vi "open fpga refs.vi"(8 "error in (no error)":errorcluster, 10 "bitfile address":path, 11 "RIO address":string) -> (0 "error out":errorcluster)   [LabVIEW 2014]
uses:
  <vilib>/NI/LVFPGA Adv Session Resources/LVFPGAAdvSessionResources.lvlib
  <vilib>/NI/LVFPGA Adv Session Resources/OpenByName.xnode
  Shared/fpga io types.ctl
  <vilib>/NI/LVFPGA Adv Session Resources/OpenByNameSubVI.vi
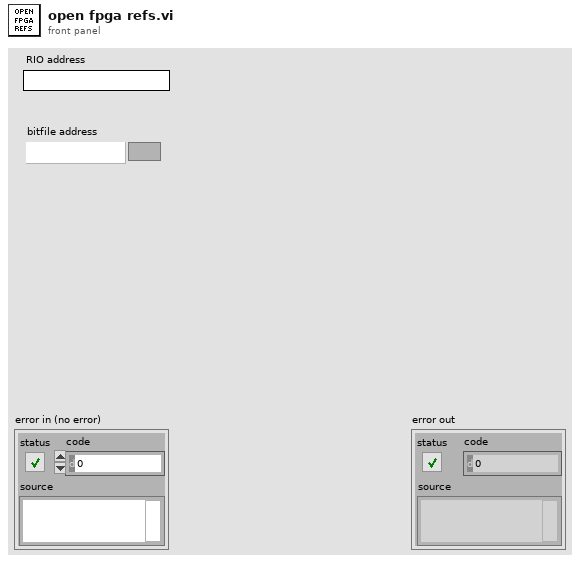
[diagram p1: front panel]
types:
  T1 = typedef "LVFPGAAdvSessionResources.lvlib/ResourceInfo.ctl" = cluster{"Resource name":string, "Data type":variant, "Resource type":enum16{"Register", "Host To Target FIFO", "Target To Host FIFO"}}
  T2 = typedef "fpga io types.ctl" = enum16{"lambda", "negate", "cal", "PWM threshold", "PWM timeout", "PWM low time", "PWM high time", "sensor model"}
  T3 = cluster{"io type":T2, "resource name":string, "channel number":i32}
  T4 = enum16{"Register", "Host To Target FIFO", "Target To Host FIFO"}
  T5 = cluster{"io type":T2, "resource name":string, "channel number":i32, "Single resource reference out":refnum<k20>}
  T6 = cluster{"Name":string, "Depth":u32, "Write? (Deprecated:Use Implementation)":bool, "Physical Channel":u32, "Base Address":u32, "Data Width":u32, "Data Type":enum32{"Boolean", "I8", "I16", "I32", "I64", "U8", "U16", "U32", "U64", "FXP", "CustomControl", "SGL"}, "FXP Properties":variant, "Write Window Address":u32, "Implementation":enum16{"niFpgaTargetToHost", "niFpgaHostToTarget", "niFpgaPeerToPeerWriter", "niFpgaPeerToPeerReader", "niCoreTargetToHost", "niCoreHostToTarget"}, "Control Set":u32}[]
  T7 = cluster{"Name":string, "type":variant, "indicator?":bool}[]
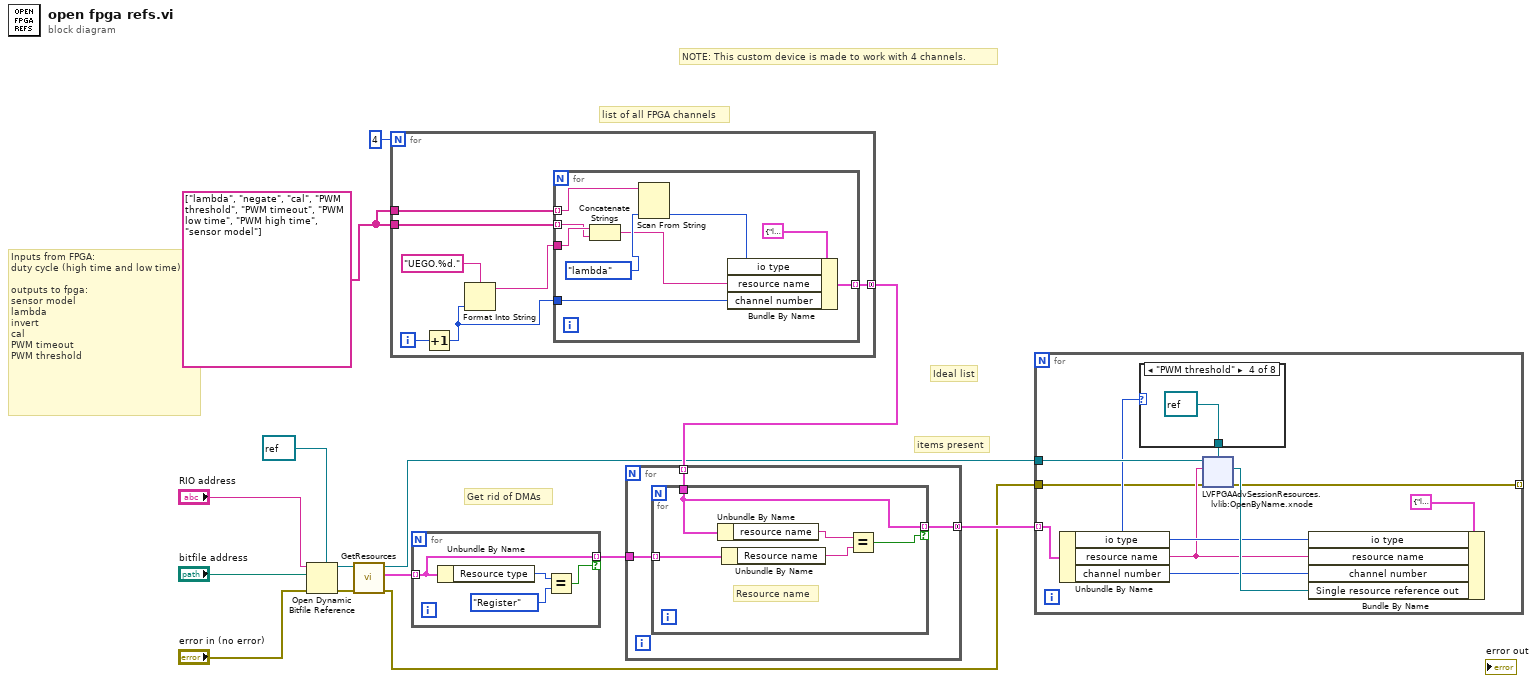
[diagram p0: block diagram]
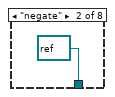
[diagram p3: hidden frame]
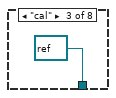
[diagram p4: hidden frame]
diagram:
  w5 = string[] ["lambda", "negate", "cal", "PWM threshold", "PWM timeout", "PWM low time", "PWM high time", "sensor model"]
  # "items present"
  # "Ideal list"
  # "NOTE: This custom device is made to work with 4 channels."
  # "list of all FPGA channels"
  # "Get rid of DMAs"
  # "Inputs from FPGA:\nduty cycle (high time and low time)\n\noutputs to fpga:\nsensor model\nlambda\ninvert\ncal\nPWM timeout\nPWM threshold"
  n1 = Open Dynamic Bitfile Reference(0:"RIO address", 1:"bitfile address", 3:"error in (no error)", 4:refnum<k20> refnum ("Type")) -> (5:w12:refnum<k20>, 8:w11:errorcluster)  [unwired: 1 in]
  n2 = call <vilib>:"GetResources.vi"("error in (no error)"=w11, "FPGA VI Reference in"=w12) -> ("error out"=w1:errorcluster, "Resource info out"=w8:T1[], "FPGA VI Reference out"=w3:refnum<k20>)  [unwired: 7 in]
  n3 = for {
    N: 4 -> [_]
    tunnel: w5 -> [w21]
    tunnel: w5 -> [w17]
    tunnel: [w15] -> w4 mode=concatenating
    i -> [w20]
    n4 = Increment(x=w20) -> (x+1=w16:i32)
    n5 = Format Into String(format string="UEGO.%d.", w16) -> (resulting string=w18:string)  [unwired: 2 in, 1 out]
    n6 = for {
      tunnel: w21 -> [w29] mode=indexing
      tunnel: w18 -> [w30]
      tunnel: w17 -> [w27] mode=indexing
      tunnel: w16 -> [w24]
      tunnel: [w22] -> w15 mode=indexing
      n7 = Concatenate Strings(w30, w29) -> (w23:string)
      n8 = Scan From String(input string=w27, default 1=fpga_io_types."lambda") -> (output 1=w25:T2)  [unwired: 3 in, 3 out]
      n9 = Bundle By Name(cluster=T3 {"io type"=enum."lambda", "resource name"="", "channel number"=0} ("output cluster"), "io type"=w25, "resource name"=w23, "channel number"=w24) -> (w22:T3)
    }
  }
  n10 = for {
    tunnel: w8 -> [w34] mode=indexing
    tunnel: [w34] -> w7 mode=indexing if=w31
    n11 = Unbundle By Name(w34) -> ("Resource type"=w33:T4)
    n12 = Equal?(x=w33, y=T4."Register" ("Resource type")) -> (x = y?=w31:bool)
  }
  n13 = for {
    tunnel: w7 -> [w37]
    tunnel: w4 -> [w36] mode=indexing
    tunnel: [w35] -> w2 mode=concatenating
    n14 = for {
      tunnel: w37 -> [w42] mode=indexing
      tunnel: [w38] -> w35 mode=indexing if=w40
      tunnel: w36 -> [w38]
      # "Resource name"
      n15 = Unbundle By Name(w38) -> ("resource name"=w39:string)
      n16 = Unbundle By Name(w42) -> ("Resource name"=w41:string)
      n17 = Equal?(x=w39, y=w41) -> (x = y?=w40:bool)
    }
  }
  n18 = for {
    tunnel: w3 -> [w52]
    tunnel: w2 -> [w51] mode=indexing
    tunnel: w1 -> [w44]
    tunnel: [w43] -> _ mode=indexing
    n19 = Unbundle By Name(w51) -> ("io type"=w47:T2, "resource name"=w45:string, "channel number"=w48:i32)
    n20 = case shown="\"PWM threshold\"" w47 {
      tunnel: [_ refnum<k20> refnum ("Single resource reference type in") refnum<k20> refnum ("Single resource reference type in") refnum<k20> refnum ("Single resource reference type in") _ _ _ _] -> w46
      frame "lambda", Default {
      }
      frame "negate" {
      }
      frame "cal" {
      }
      frame "PWM threshold" {
      }
      frame "PWM timeout" {
      }
      frame "PWM low time" {
      }
      frame "PWM high time" {
      }
      frame "sensor model" {
      }
    }
    n21 = xnode "LVFPGAAdvSessionResources.lvlib:OpenByName.xnode"("FPGA VI Reference in"=w52, "Resource name in"=w45, "Single resource reference type in"=w46, "Error in"=w44) -> ("Single resource reference out"=w49:refnum<k20>, "Error out"=w43:errorcluster)  [unwired: 1 out]
    n22 = Bundle By Name(cluster=T5 {"io type"=enum."lambda", "resource name"="", "channel number"=0, "Single resource reference out"=refnum} ("output cluster"), "io type"=w47, "resource name"=w45, "channel number"=w48, "Single resource reference out"=w49) -> ()  [unwired: 1 out]
  }
